vi "Global - VISA.vi"() -> ()   [LabVIEW 2019]
panel:
  in  "VISA":refnum<visa-resource-name>[](array[refnum])
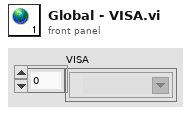
[diagram p1: front panel]
diagram:
